vi "Read VI name.vi"(8 "error in":errorcluster, 11 "io configuration in":refnum<class "io configuration.lvclass">) -> (0 "error out":errorcluster, 2 "VI name":string, 3 "io configuration out":refnum<class "io configuration.lvclass">)   [LabVIEW 2015, in "io configuration.lvclass"]
uses:
  io configuration.lvclass
  io configuration.lvclass/io configuration.ctl
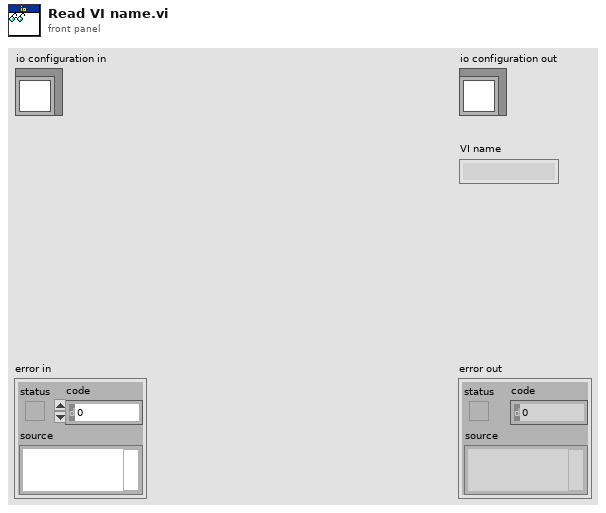
[diagram p1: front panel]
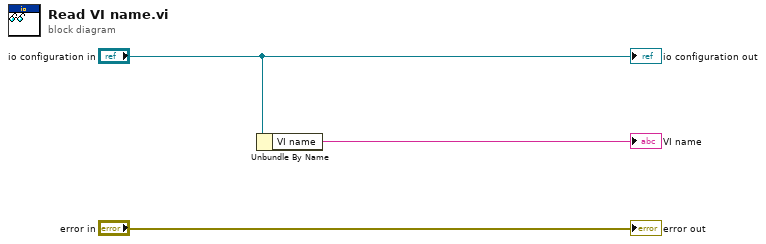
[diagram p0: block diagram]
diagram:
  n1 = Unbundle By Name("io configuration in") -> ("VI name"=→"VI name":string)
  "error out" <- "error in"
  "io configuration out" <- "io configuration in"
